vi "Update status--value--default format.vi"(8 "error in (no error)":errorcluster, 11 "String Value":string) -> (0 "error out":errorcluster)   [LabVIEW 2018, in "status_text_indicator.lvlib"]
uses:
  status_text_indicator.lvlib
  PTRL/String_Control/string_control.lvlib
panel:
  # "Development\ncontrols/indicators useful for development and testing, but which are not outputs of the VI"
  # "Input\nInputs to the VI"
  # "Output\nOutputs of the VI"
  # "Description\n\nBlank VI with error handling case. \n\nSummarize the use of this VI in this space."
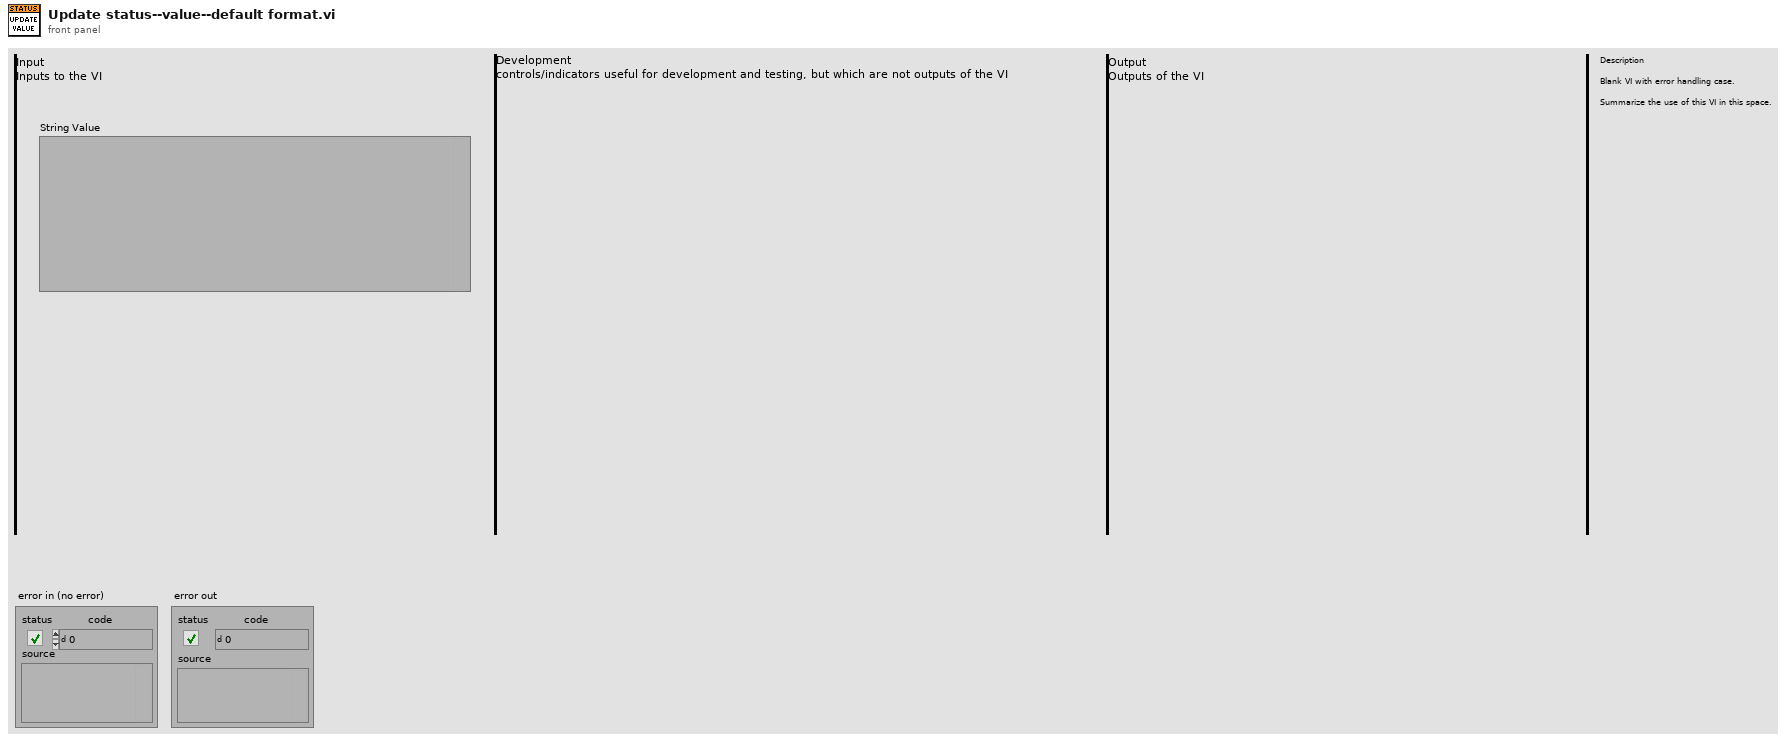
[diagram p1: front panel]
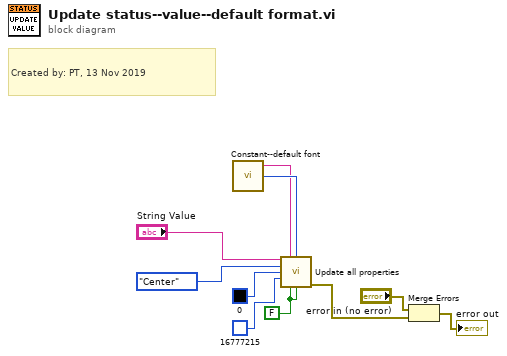
[diagram p0: block diagram]
diagram:
  w7 = FALSE ("Bold? [Default = False]")
  # "Created by: PT, 13 Nov 2019"
  n1 = call "Constant--default font.vi"() -> ("Font size"=w6:u32, "Font name"=w5:string)  [unwired: 1 in]
  n2 = call "Update all properties.vi"("String Value  [Default = \"\" (blank)]"="String Value", "Font Name [Default = \"Application Font\"]"=w5, "Font size [Default = 15]"=w6, "Justification [Default = Left]"=enum16{"Left", "Center", "Right"}."Center", "Text Colour [Default=Pure Black=(0,0,0)]"=u32 0 ("Background color"), "Background Colour [Default=Pure White=(255,255,255)]"=u32 16777215 ("Text color"), "Bold? [Default = False]"=w7, "Italic? [Default = False]"=w7) -> ("error out"=w8:errorcluster)  [unwired: 7 in]
  n3 = Merge Errors("error in (no error)", w8) -> (→"error out":errorcluster)
